vi "DigitalOutputSetLEDForwardVoltage.vi"(0 "error in (no error)":errorcluster, 2 "LEDForwardVoltage":u32(ring)=7 items=["LED_FORWARD_VOLTAGE_1_7V"=1, "LED_FORWARD_VOLTAGE_2_75V"=2, "LED_FORWARD_VOLTAGE_3_2V"=3, "LED_FORWARD_VOLTAGE_3_9V"=4, "LED_FORWARD_VOLTAGE_4_0V"=5, "LED_FORWARD_VOLTAGE_4_8V"=6, "LED_FORWARD_VOLTAGE_5_0V"=7, "LED_FORWARD_VOLTAGE_5_6V"=8], 3 "Device In":u64) -> (7 "error out":errorcluster, 10 "Device Out":u64)   [LabVIEW 2020, in "Phidget Digital Output.lvlib"]
doc: "${LEDForwardVoltage:Header}"
uses:
  <instrlib>/Phidgets/Phidget Digital Output/Phidget Digital Output.lvlib
  <instrlib>/Phidgets/Phidget Common/Phidget Common.lvlib
  phidget22.dll
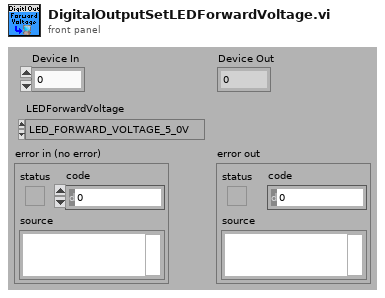
[diagram p1: front panel]
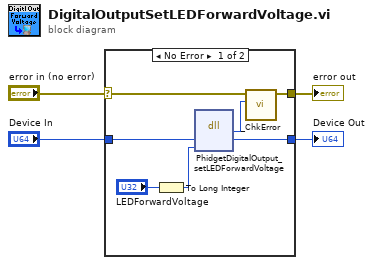
[diagram p0: block diagram]
diagram:
  n1 = case shown="No Error" "error in (no error)" {
    selector: "error in (no error)" -> [w9 w13]
    tunnel: [w8 w13] -> w3
    tunnel: "Device In" -> [w11 w12]
    tunnel: [w10 w12] -> w1
    frame No Error {
      n2 = To Long Integer(number="LEDForwardVoltage") -> (32bit integer=w6:i32)
      n3 = dll-call lib="phidget22.dll" fn="PhidgetDigitalOutput_setLEDForwardVoltage"("phid"=w11, "trigger"=w6) -> ("return type"=w7:i32, "phid"=w10:u64)  [unwired: 4 in, 2 out]
      n4 = call <instrlib>:"_ChkError.vi"("Return Code"=w7, "error in (no error)"=w9) -> ("error out"=w8:errorcluster)  [unwired: 9 in]
    }
    frame Error {
    }
  }
  "error out" <- w3
  "Device Out" <- w1
